vi "Control - GDI - Cranking.vi"(0 "Control Inputs":T4={"Engine Speed [RPM]"=0.0, "Engine Status"=enum."STALLED", "Load Control \nMode"=enum."High-Idle Governor", "dt(s)"=0.0, "Number of Cylinders"=0, "Engine Displacement [cc]"=0.0, "StoichAFR"=0.0, "Q.LHV Fuel [kJ/kg]"=0.0, "BattV PSU [V]"=0.0, "12V PSU [V]"=0.0, "5V PSU [V]"=0.0, "Pedal Position [%]"=0.0, "Oil Pressure [kPa]"=0.0, "Oil Temp [C]"=0.0, "Oil Level [%]"=0.0, "Engine Coolant Temp (ECT) [C]"=0.0, "Engine Coolant Pressure [kPa]"=0.0, "Rail Pressure [bar]"=0.0, "Fuel Pressure [kPa]"=0.0, "Fuel Temp [C]"=0.0, "Vacuum Pressure [kPa]"=0.0, "Throttle Position [%]"=0.0, "Cam1 Advance [CAD]"=0.0, "Cam2 Advance [CAD]"=0.0, "Cam3 Advance [CAD]"=0.0, "Cam4 Advance [CAD]"=0.0, "CA50 Control Output [CAD]"=[], "CA50 Control Output Valid"=[], "Intake Air Temp (IAT) [C]"=0.0, "Barometric Air Pressure [kPa]"=0.0, "Intake Air Rel. Humidity [%]"=0.0, "Mass Air Flow (MAF) [kg/hr]"=0.0, "Turbo Inlet Air Pressure [kPa]"=0.0, "Turbo Inlet Air Temp [C]"=0.0, "Turbo Outlet Air Pressure [kPa]"=0.0, "Turbo Outlet Air Temp [C]"=0.0, "CAC Outlet Pressure [kPa]"=0.0, "CAC Outlet Temp [C]"=0.0, "Intake Manifold Pressure (MAP) [kPa]"=0.0, "Intake Manifold Temp (MAT) [C]"=0.0, "Exhaust Manifold Pressure [kPa]"=0.0, "Exhaust Manifold Temp [C]"=0.0, "HighP EGR Cooler Outlet Pressure [kPa]"=0.0, "HighP EGR Cooler Outlet Temp [C]"=0.0, "HighP EGR Differential Pressure [kPa]"=0.0, "HighP EGR Valve Position [%]"=0.0, "Turbo Outlet Exhaust Pressure [kPa]"=0.0, "Turbo Outlet Exhaust Temp [C]"=0.0, "VGT Position 1 [%]"=0.0, "VGT Position 2 [%]"=0.0, "Turbo Speed 1 [RPM]"=0.0, "Turbo Speed 2 [RPM]"=0.0, "LowP EGR Differential Pressure [kPa]"=0.0, "LowP EGR Valve Position [%]"=0.0, "UEGO1Lambda"=0.0, "UEGO1_Hot"=FALSE, "UEGO2Lambda"=0.0, "UEGO2_Hot"=FALSE, "Knock Intensity"=[], "Knock"=[]} {"Knock Intensity" format="%.2f"; "CA50 Control Output [CAD]" format="%.2f"; "Exhaust Manifold Temp [C]" format="%#_6f"; "UEGO2Lambda" format="%.2f"; "Intake Manifold Temp (MAT) [C]" format="%#_6f"; "UEGO1Lambda" format="%.2f"}, 1 "Available Air Mass [mg/cyc]":sgl, 5 "Control Outputs In":T1) -> (19 "Control Outputs":T1)   [LabVIEW 2015, in "ECS-RT.lvlib"]
uses:
  ECS-RT.lvlib
  Typedefs/Control Inputs/Control Inputs.ctl
  Typedefs/EPT/Engine Status.ctl
  Typedefs/MISC/Load Control Mode.ctl
  Typedefs/Control Outputs/Control Outputs.ctl
  Typedefs/Control Outputs/Injection Quantity.ctl
  Typedefs/Control Outputs/Injection Timing.ctl
  ECS-Shared.lvlib
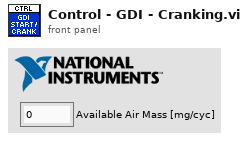
[diagram p1: front panel]
types:
  T1 = typedef "ECS-Shared.lvlib/Control Outputs.ctl" = cluster{"Pedal Desired [%]":sgl, "MEP Desired [bar]":sgl, "Fuel Desired [mg/cyc]":sgl, "Intake MAP Desired [kPa]":sgl, "Cam1 Advance Setpoint [CAD]":sgl, "Cam2 Advance Setpoint [CAD]":sgl, "HighP EGR Position Setpoint [%Open]":sgl, "LowP EGR Position Setpoint [%Open]":sgl, "Rail Pressure Setpoint [bar]":sgl, "Wastegate1 Position Setpoint [%Open]":sgl, "Wastegate2 Position Setpoint [%Open]":sgl, "VGT1 Position Setpoint [%Open]":sgl, "VGT2 Position Setpoint [%Open]":sgl, "Throttle1 Position Setpoint [%Open]":sgl, "Throttle2 Position Setpoint [%Open]":sgl, "TurboBPV Position Setpoint [%Open]":sgl, "Spark Dwells [msec]":sgl[], "Spark Timings [DBTDC]":sgl[], "PFI Quantities [mg/inj]":sgl[], "PFI Timings [DBTDC]":sgl[], "DI Quantities [mg/inj]":T2[], "DI Timings [DBTDC]":T3[]}
  T2 = typedef "ECS-Shared.lvlib/Injection Quantity.ctl" = cluster{"Pilot1Quantity [mg/inj]":sgl, "Pilot2Quantity [mg/inj]":sgl, "MainQuantity [mg/inj]":sgl, "Post1Quantity [mg/inj]":sgl, "Post2Quantity [mg/inj]":sgl}
  T3 = typedef "ECS-Shared.lvlib/Injection Timing.ctl" = cluster{"Pilot1SOI [DBTDC]":sgl, "Pilot2SOI [DBTDC]":sgl, "MainSOI [DBTDC]":sgl, "Post1SOI [DBTDC]":sgl, "Post2SOI [DBTDC]":sgl}
  T4 = typedef "ECS-Shared.lvlib/Control Inputs.ctl" = cluster{"Engine Speed [RPM]":sgl, "Engine Status":T5, "Load Control \nMode":T6, "dt(s)":sgl, "Number of Cylinders":u8, "Engine Displacement [cc]":sgl, "StoichAFR":sgl, "Q.LHV Fuel [kJ/kg]":sgl, "BattV PSU [V]":sgl, "12V PSU [V]":sgl, "5V PSU [V]":sgl, "Pedal Position [%]":sgl, "Oil Pressure [kPa]":sgl, "Oil Temp [C]":sgl, "Oil Level [%]":sgl, "Engine Coolant Temp (ECT) [C]":sgl, "Engine Coolant Pressure [kPa]":sgl, "Rail Pressure [bar]":sgl, "Fuel Pressure [kPa]":sgl, "Fuel Temp [C]":sgl, "Vacuum Pressure [kPa]":sgl, "Throttle Position [%]":sgl, "Cam1 Advance [CAD]":sgl, "Cam2 Advance [CAD]":sgl, "Cam3 Advance [CAD]":sgl, "Cam4 Advance [CAD]":sgl, "CA50 Control Output [CAD]":sgl[], "CA50 Control Output Valid":bool[], "Intake Air Temp (IAT) [C]":sgl, "Barometric Air Pressure [kPa]":sgl, "Intake Air Rel. Humidity [%]":sgl, "Mass Air Flow (MAF) [kg/hr]":sgl, "Turbo Inlet Air Pressure [kPa]":sgl, "Turbo Inlet Air Temp [C]":sgl, "Turbo Outlet Air Pressure [kPa]":sgl, "Turbo Outlet Air Temp [C]":sgl, "CAC Outlet Pressure [kPa]":sgl, "CAC Outlet Temp [C]":sgl, "Intake Manifold Pressure (MAP) [kPa]":sgl, "Intake Manifold Temp (MAT) [C]":sgl, "Exhaust Manifold Pressure [kPa]":sgl, "Exhaust Manifold Temp [C]":sgl, "HighP EGR Cooler Outlet Pressure [kPa]":sgl, "HighP EGR Cooler Outlet Temp [C]":sgl, "HighP EGR Differential Pressure [kPa]":sgl, "HighP EGR Valve Position [%]":sgl, "Turbo Outlet Exhaust Pressure [kPa]":sgl, "Turbo Outlet Exhaust Temp [C]":sgl, "VGT Position 1 [%]":sgl, "VGT Position 2 [%]":sgl, "Turbo Speed 1 [RPM]":sgl, "Turbo Speed 2 [RPM]":sgl, "LowP EGR Differential Pressure [kPa]":sgl, "LowP EGR Valve Position [%]":sgl, "UEGO1Lambda":sgl, "UEGO1_Hot":bool, "UEGO2Lambda":sgl, "UEGO2_Hot":bool, "Knock Intensity":sgl[], "Knock":bool[]}
  T5 = typedef "ECS-Shared.lvlib/Engine Status.ctl" = enum16{"OFF", "STALLED", "CRANKING", "RUNNING", "ACCEL", "DECEL", "SAFE"}
  T6 = typedef "ECS-Shared.lvlib/Load Control Mode.ctl" = enum16{"No Governor", "Low-Idle Governor", "High-Idle Governor"}
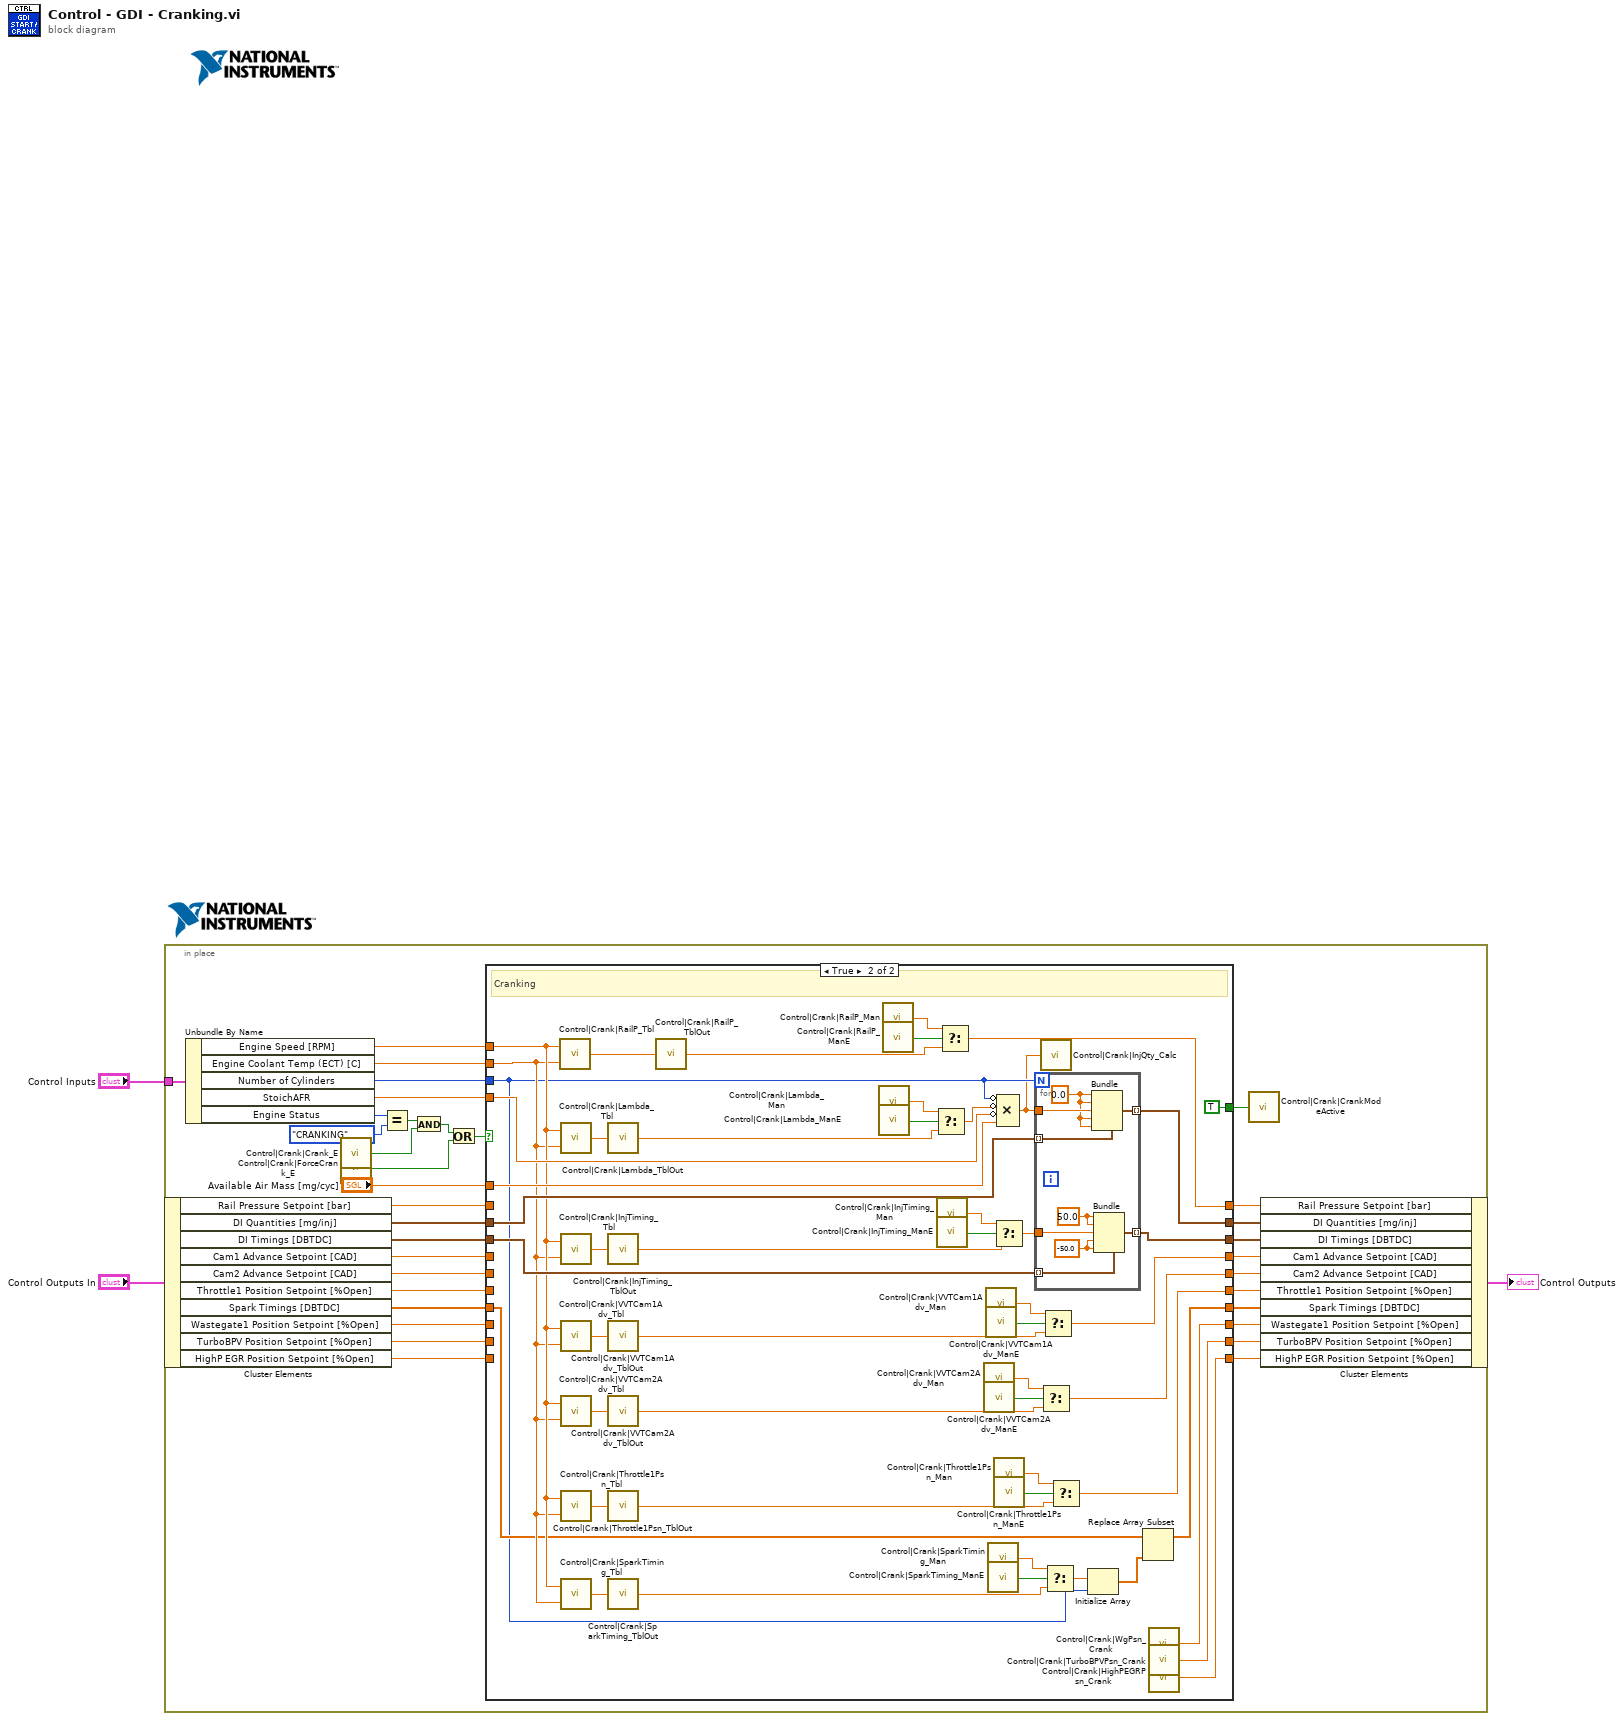
[diagram p0: block diagram]
diagram:
  n1 = in-place {
    in-place-border: "Control Inputs" -> [w33]
    n2 = in-place-cluster #1("Control Outputs In") -> ("Rail Pressure Setpoint [bar]"=w15:sgl, "DI Quantities [mg/inj]"=w16:T2[], "DI Timings [DBTDC]"=w17:T3[], "Cam1 Advance Setpoint [CAD]"=w18:sgl, "Cam2 Advance Setpoint [CAD]"=w19:sgl, "Throttle1 Position Setpoint [%Open]"=w20:sgl, "Spark Timings [DBTDC]"=w5:sgl[], "Wastegate1 Position Setpoint [%Open]"=w21:sgl, "TurboBPV Position Setpoint [%Open]"=w22:sgl, "HighP EGR Position Setpoint [%Open]"=w23:sgl)
    n3 = Unbundle By Name(w33) -> ("Engine Speed [RPM]"=w37:sgl, "Engine Coolant Temp (ECT) [C]"=w36:sgl, "Number of Cylinders"=w35:u8, "StoichAFR"=w34:sgl, "Engine Status"=w31:T5)
    n4 = call "Control|Crank|Crank_E"() -> ("Value"=w28:bool)
    n5 = call "Control|Crank|ForceCrank_E"() -> ("Value"=w26:bool)
    n6 = Equal?(x=w31, y=Engine_Status."CRANKING" ("Engine Status")) -> (x = y?=w29:bool)
    n7 = And(x=w29, y=w28) -> (x .and. y?=w25:bool)
    n8 = Or(x=w25, y=w26) -> (x .or. y?=w27:bool)
    n9 = case shown="True" w27 {
      tunnel: w37 -> [_ w55]
      tunnel: w36 -> [_ w54]
      tunnel: w35 -> [_ w51]
      tunnel: w34 -> [_ w71]
      tunnel: "Available Air Mass [mg/cyc]" -> [_ w70]
      tunnel: [_ TRUE] -> w32
      tunnel: w23 -> [w39 _]
      tunnel: w22 -> [w40 _]
      tunnel: w21 -> [w41 _]
      tunnel: w20 -> [w42 _]
      tunnel: w19 -> [w43 _]
      tunnel: w18 -> [w44 _]
      tunnel: w17 -> [w45 w68]
      tunnel: w16 -> [w46 w69]
      tunnel: w15 -> [w47 _]
      tunnel: [w47 w79] -> w14
      tunnel: [w46 w63] -> w13
      tunnel: [w45 w62] -> w12
      tunnel: [w44 w58] -> w11
      tunnel: [w43 w57] -> w10
      tunnel: [w42 w56] -> w9
      tunnel: [w41 w76] -> w8
      tunnel: [w40 w77] -> w7
      tunnel: [w39 w78] -> w6
      tunnel: w5 -> [w38 w53]
      tunnel: [w38 w49] -> w4
      frame False {
        # "Normal Operation"
      }
      frame True {
        # "Cranking"
        n10 = call "Control|Crank|RailP_Tbl"("Y Index"=w54, "X Index"=w55) -> ("Z"=w80:sgl)
        n11 = call "Control|Crank|Lambda_Tbl"("Y Index"=w54, "X Index"=w55) -> ("Z"=w73:sgl)
        n12 = call "Control|Crank|InjTiming_Tbl"("Y Index"=w54, "X Index"=w55) -> ("Z"=w67:sgl)
        n13 = call "Control|Crank|VVTCam1Adv_Tbl"("Y Index"=w54, "X Index"=w55) -> ("Z"=w59:sgl)
        n14 = call "Control|Crank|VVTCam2Adv_Tbl"("Y Index"=w54, "X Index"=w55) -> ("Z"=w88:sgl)
        n15 = call "Control|Crank|Throttle1Psn_Tbl"("Y Index"=w54, "X Index"=w55) -> ("Z"=w89:sgl)
        n16 = call "Control|Crank|SparkTiming_Tbl"("Y Index"=w54, "X Index"=w55) -> ("Z"=w85:sgl)
        n17 = call "Control|Crank|Lambda_TblOut"("Value"=w73) -> ()
        n18 = call "Control|Crank|InjTiming_TblOut"("Value"=w67) -> ()
        n19 = call "Control|Crank|VVTCam1Adv_TblOut"("Value"=w59) -> ()
        n20 = call "Control|Crank|VVTCam2Adv_TblOut"("Value"=w88) -> ()
        n21 = call "Control|Crank|Throttle1Psn_TblOut"("Value"=w89) -> ()
        n22 = call "Control|Crank|SparkTiming_TblOut"("Value"=w85) -> ()
        n23 = call "Control|Crank|RailP_TblOut"("Value"=w80) -> ()
        n24 = call "Control|Crank|Lambda_Man"() -> ("Value"=w75:sgl)
        n25 = call "Control|Crank|Lambda_ManE"() -> ("Value"=w74:bool)
        n26 = call "Control|Crank|RailP_Man"() -> ("Value"=w82:sgl)
        n27 = call "Control|Crank|RailP_ManE"() -> ("Value"=w81:bool)
        n28 = Select(t=w75, s=w74, f=w73) -> (s? t:f=w72:sgl)
        n29 = call "Control|Crank|InjTiming_Man"() -> ("Value"=w66:sgl)
        n30 = call "Control|Crank|InjTiming_ManE"() -> ("Value"=w65:bool)
        n31 = Select(t=w82, s=w81, f=w80) -> (s? t:f=w79:sgl)
        n32 = call "Control|Crank|VVTCam2Adv_Man"() -> ("Value"=w86:sgl)
        n33 = call "Control|Crank|VVTCam2Adv_ManE"() -> ("Value"=w87:bool)
        n34 = call "Control|Crank|VVTCam1Adv_Man"() -> ("Value"=w61:sgl)
        n35 = call "Control|Crank|VVTCam1Adv_ManE"() -> ("Value"=w60:bool)
        n36 = call "Control|Crank|SparkTiming_Man"() -> ("Value"=w84:sgl)
        n37 = call "Control|Crank|SparkTiming_ManE"() -> ("Value"=w83:bool)
        n38 = Select(t=w66, s=w65, f=w67) -> (s? t:f=w64:sgl)
        n39 = call "Control|Crank|Throttle1Psn_Man"() -> ("Value"=w91:sgl)
        n40 = call "Control|Crank|Throttle1Psn_ManE"() -> ("Value"=w90:bool)
        n41 = Compound Arithmetic op=MULTIPLY(invert w51, invert w72, invert w71, w70) -> (w48:dbl)
        n42 = for {
          N: w51 -> [_]
          tunnel: [w101] -> w63 mode=indexing
          tunnel: w69 -> [w100] mode=indexing
          tunnel: w48 -> [w99]
          tunnel: w64 -> [w95]
          tunnel: [w94] -> w62 mode=indexing
          tunnel: w68 -> [w93] mode=indexing
          w97 = sgl -50.0 ("Pilot1SOI [DBTDC]")
          w96 = sgl 50.0 ("Pilot1SOI [DBTDC]")
          w98 = sgl 0.0 ("Pilot1Quantity [mg/inj]")
          n43 = Bundle(cluster=w100, "Pilot1Quantity [mg/inj]"=w98, "Pilot2Quantity [mg/inj]"=w98, "MainQuantity [mg/inj]"=w99, "Post1Quantity [mg/inj]"=w98, "Post2Quantity [mg/inj]"=w98) -> (w101:T2)
          n44 = Bundle(cluster=w93, "Pilot1SOI [DBTDC]"=w96, "Pilot2SOI [DBTDC]"=w96, "MainSOI [DBTDC]"=w95, "Post1SOI [DBTDC]"=w97, "Post2SOI [DBTDC]"=w97) -> (w94:T3)
        }
        n45 = call "Control|Crank|InjQty_Calc"("Value"=w48) -> ()
        n46 = Select(t=w86, s=w87, f=w88) -> (s? t:f=w57:sgl)
        n47 = Select(t=w61, s=w60, f=w59) -> (s? t:f=w58:sgl)
        n48 = Select(t=w84, s=w83, f=w85) -> (s? t:f=w52:sgl)
        n49 = Select(t=w91, s=w90, f=w89) -> (s? t:f=w56:sgl)
        n50 = Initialize Array(w52, w51) -> (w50:sgl[])
        n51 = Replace Array Subset(array=w53, new element=w50) -> (w49:sgl[])  [unwired: 1 in]
        n52 = call "Control|Crank|WgPsn_Crank"() -> ("Value"=w76:sgl)
        n53 = call "Control|Crank|TurboBPVPsn_Crank"() -> ("Value"=w77:sgl)
        n54 = call "Control|Crank|HighPEGRPsn_Crank"() -> ("Value"=w78:sgl)
      }
    }
    n55 = call "Control|Crank|CrankModeActive"("Value"=w32) -> ()
    n56 = in-place-cluster #1("Rail Pressure Setpoint [bar]"=w14, "DI Quantities [mg/inj]"=w13, "DI Timings [DBTDC]"=w12, "Cam1 Advance Setpoint [CAD]"=w11, "Cam2 Advance Setpoint [CAD]"=w10, "Throttle1 Position Setpoint [%Open]"=w9, "Spark Timings [DBTDC]"=w4, "Wastegate1 Position Setpoint [%Open]"=w8, "TurboBPV Position Setpoint [%Open]"=w7, "HighP EGR Position Setpoint [%Open]"=w6) -> (→"Control Outputs":T1)
  }
